vi "BioFeedbackEMG.vi"(10 "stop":bool, 11 "Start":bool) -> (2 "filtered signal (single sample)":waveform(dbl)(graph), 3 "Data Levels":dbl(slide) scale=0.0..0.07)   [LabVIEW 2016]
uses:
  <vilib>/Analysis/NI_AALPro.lvlib
  <vilib>/Analysis/5stat.llb/RMS (DBL).vi
panel:
  in  "Device":u32
  in  "Sample Duratiopn":dbl
  in  "Trial":dbl
  out "(INTERNAL) Buffer Array Size":i32
  out "(INTERNAL) Buffer Index":i32
  out "smooth":dynamicdata(graph)
  out "Thermometer Elapsed Frames":i32
  in  "Thermometer\nFps":dbl
  out "AggregateSignalData":waveform(dbl)[](array[waveform])
  out "rms data":dbl(graph)
  out "Moving Average Length (s)":dbl
  in  "Sample rate (Hz)":dbl=22050.0
  in  "Lower Cut-Off (Hz)":dbl=20.0 caption="Lower Cut-Off"
  in  "Upper Cut-Off (Hz)":dbl=300.0 caption="Upper Cut-Off"
  out "aggregate signal":waveform(dbl)[](graph)
  in  "Number of Samples in\n Moving Average":dbl
  # "Biofeedback"
  # "Internal"
  # "Settings"
  # "Filter Settings"
  # "Bandpass Filter"
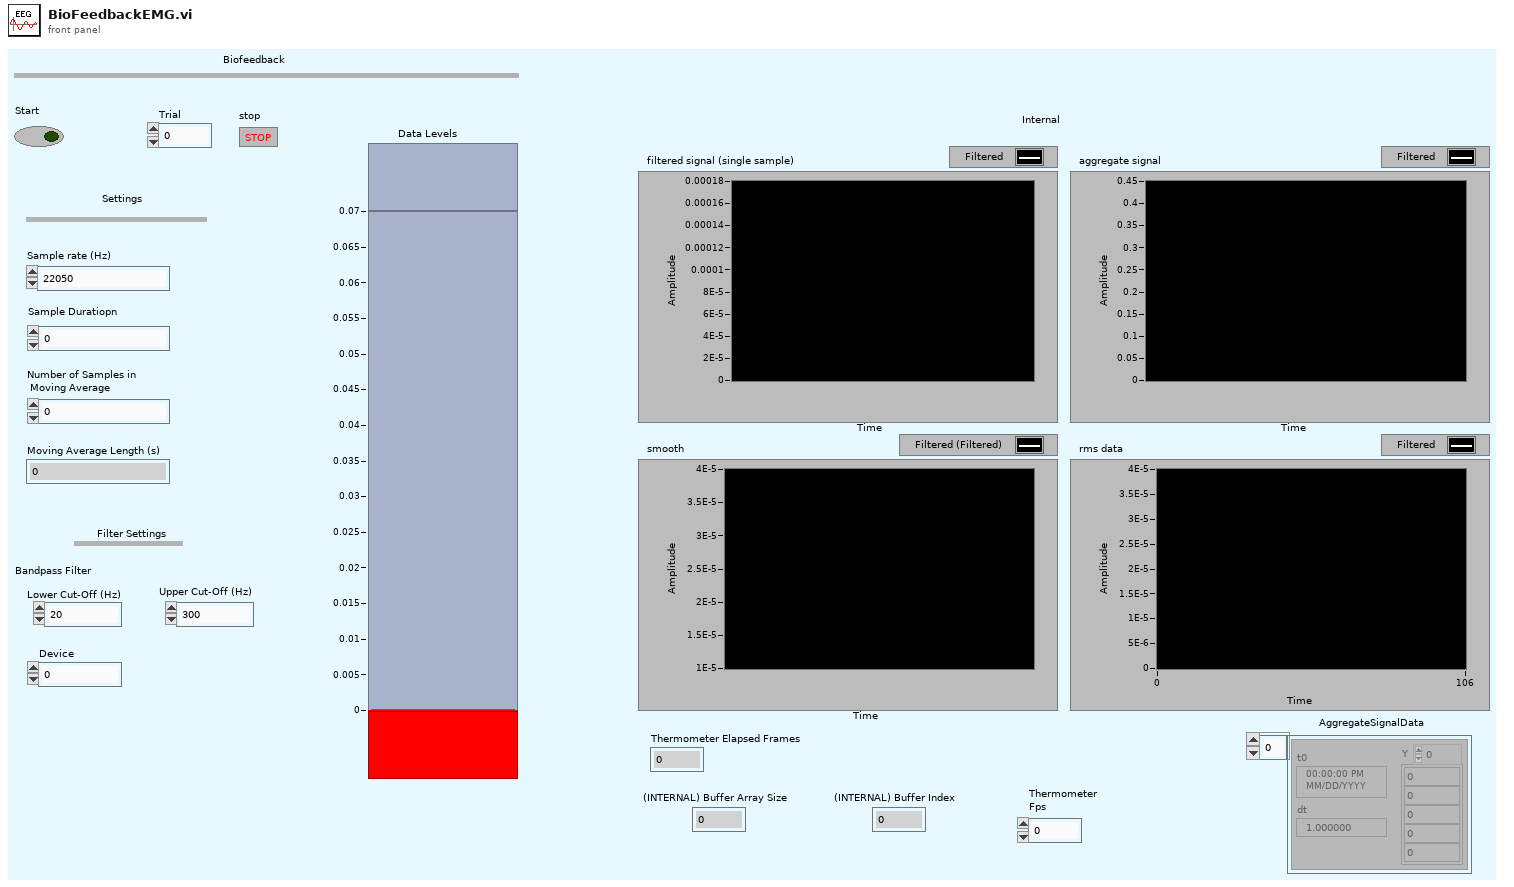
[diagram p1: front panel]
types:
  T1 = typedef "WaveformArrayControl.ctl" = waveform(dbl)[]
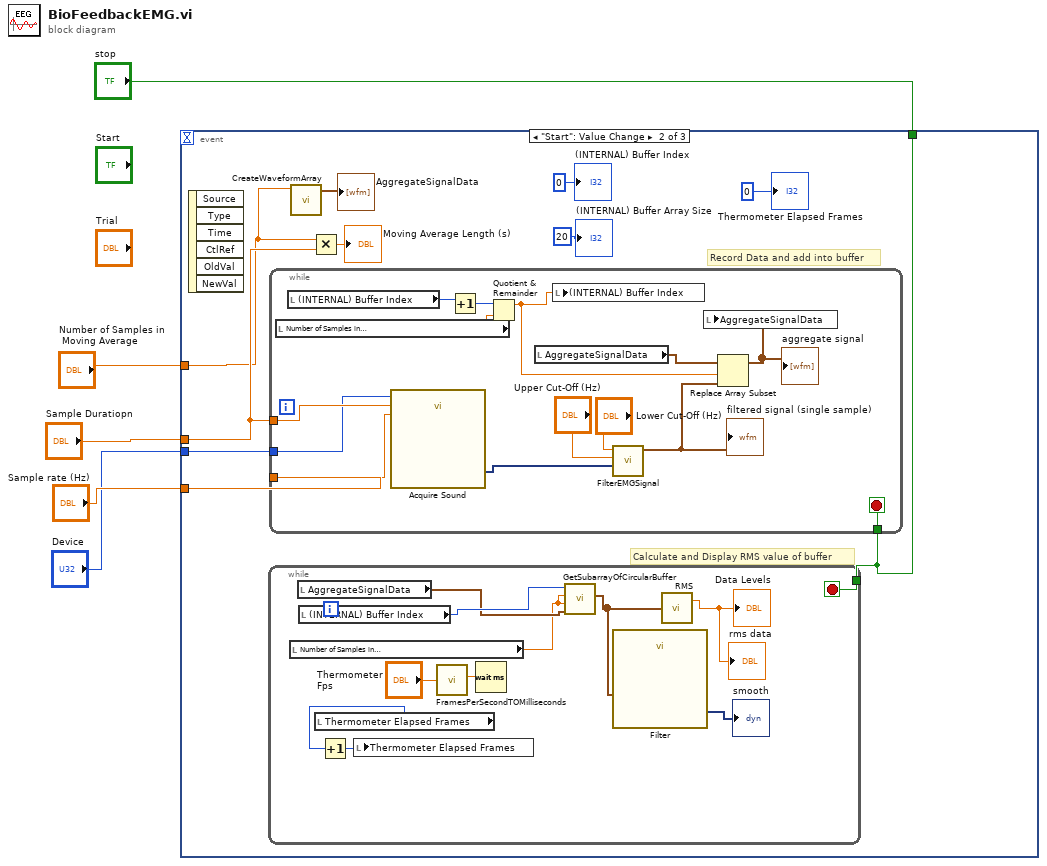
[diagram p0: block diagram]
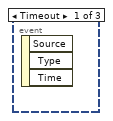
[diagram p2: hidden frame]
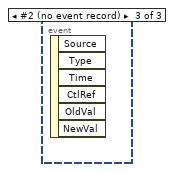
[diagram p3: hidden frame]
diagram:
  n1 = event shown="[1] \"Start\": Value Change" {
    selector: _ -> [_ _ _]
    dyn-events: _ -> [_ _ _]
    timeout: _ -> [_ _ _]
    tunnel: "Number of Samples in\n Moving Average" -> [_ w8 _]
    tunnel: "Sample Duratiopn" -> [_ w10 _]
    tunnel: "Sample rate (Hz)" -> [_ w9 _]
    tunnel: "stop" -> [_ w7 _]
    tunnel: "Device" -> [_ w6 _]
    event Timeout {
      n2 = event-data() -> ()  [unwired: 1 in, 3 out]
    }
    event "Start": Value Change {
      # "Record Data and add into buffer"
      # "Calculate and Display RMS value of buffer"
      n3 = event-data() -> ()  [unwired: 1 in, 6 out]
      n4 = while {
        tunnel: w7 -> [w26]
        stop <- w26 stop-if-true
        n5 = local read "Number of Samples in\n Moving Average"() -> (w16:dbl)
        n6 = local read "AggregateSignalData"() -> (w19:waveform(dbl)[])
        n7 = local read "(INTERNAL) Buffer Index"() -> (w20:i32)
        n8 = local read "Thermometer Elapsed Frames"() -> (w23:i32)
        n9 = Increment(x=w23) -> (x+1=w22:i32)
        n10 = local write "Thermometer Elapsed Frames"(w22) -> ()
        n11 = call "FramesPerSecondTOMilliseconds.vi"("Thermometer\nFps"="Thermometer\nFps") -> ("x*y"=w24:dbl)  [unwired: 10 in]
        n12 = Wait (ms)(milliseconds to wait=w24) -> ()  [unwired: 1 out]
        n13 = call "GetSubarrayOfCircularBuffer.vi"("initialized array"=w19, "buffer size"=w16, "subset size"=w16, "start index"=w20) -> ("initialized array 2"=w18:T1)  [unwired: 7 in]
        n14 = call "Filter"("Signal"=w18) -> ("Filtered Signal"=→"smooth":dynamicdata)  [unwired: 9 in, 1 out]
        n15 = call-poly <vilib>:"RMS.vi"("X"=w18) -> ("rms value"=→"Data Levels" →"rms data":dbl)  [unwired: 1 out]
      }
      n16 = while {
        tunnel: w7 -> [w38]
        tunnel: w10 -> [w29]
        tunnel: w9 -> [w28]
        tunnel: w6 -> [w27]
        stop <- w38 stop-if-true
        n17 = local read "Number of Samples in\n Moving Average"() -> (w32:dbl)
        n18 = local read "(INTERNAL) Buffer Index"() -> (w34:i32)
        n19 = call "Acquire Sound"("Device"=w27, "Duration (s)"=w29, "Sample rate (Hz)"=w28) -> ("Data"=w31:dynamicdata)  [unwired: 15 in, 1 out]
        n20 = Increment(x=w34) -> (x+1=w33:i32)
        n21 = Quotient & Remainder(x=w33, y=w32) -> (x-y*floor(x/y)=w30:dbl)  [unwired: 1 out]
        n22 = local read "AggregateSignalData"() -> (w36:waveform(dbl)[])
        n23 = local write "(INTERNAL) Buffer Index"(w30) -> ()
        n24 = call "FilterEMGSignal.vi"("Data"=w31, "Upper Cut-Off"="Upper Cut-Off (Hz)", "Lower Cut-Off"="Lower Cut-Off (Hz)") -> ("Waveform"=w37:waveform(dbl))  [unwired: 8 in]
        "filtered signal (single sample)" <- w37
        n25 = Replace Array Subset(array=w36, new element=w37, index=w30) -> (w35:waveform(dbl)[])
        "aggregate signal" <- w35
        n26 = local write "AggregateSignalData"(w35) -> ()
      }
      n27 = call "CreateWaveformArray.vi"("bufferSize"=w8) -> ("initialized array"=→"AggregateSignalData":waveform(dbl)[])  [unwired: 10 in]
      n28 = Multiply(x=w8, y=w10) -> (x*y=→"Moving Average Length (s)":dbl)
      "Thermometer Elapsed Frames" <- 0 ("Thermometer Elapsed Frames")
      "(INTERNAL) Buffer Index" <- 0 ("Current Buffer Index")
      "(INTERNAL) Buffer Array Size" <- 20 ("(INTERNAL) Buffer Array Size")
    }
    event #2 (no event record) {
      n29 = event-data() -> ()  [unwired: 1 in, 6 out]
    }
  }
